vi "ED_Initialize.vi"(4 "error in (no error)":errorcluster, 6 "IP address":string="192.168.0.10") -> (0 "error out":errorcluster, 3 "connection ID":refnum<k5>)   [LabVIEW 2020, in "CAENels EASY-DRIVER.lvlib"]
doc: "Initializes the connection with the EASY-DRIVER module at the specified IP address."
uses:
  CAENels EASY-DRIVER.lvlib
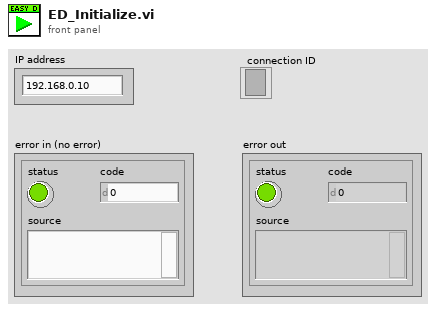
[diagram p1: front panel]
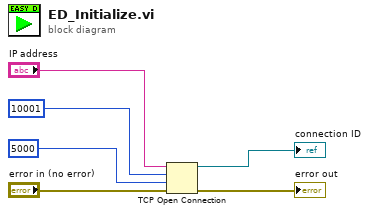
[diagram p0: block diagram]
diagram:
  n1 = TCP Open Connection(address="IP address", remote port or service name=u16 10001, timeout ms (60000)=5000, error in (no error)="error in (no error)") -> (connection ID=→"connection ID":refnum<k5>, error out=→"error out":errorcluster)  [unwired: 1 in]
